vi "CvrtCell2Data.vi"(8 "error in (no error)":errorcluster, 9 "ge_HdrNames":T1, 10 "Item Name":string, 11 "RTD in":refnum<class "RTD.lvclass">) -> (0 "error out":errorcluster, 3 "RTD out":refnum<class "RTD.lvclass">)   [LabVIEW 2018, in "Measurement Channels.lvlib" / "RTD.lvclass"]
uses:
  RTD.lvclass
  C:/Users/Jeff Tipps/Documents/DAQMan/source/Classes/Measurements/Class Channel/Channel.lvclass
  Common/Controls/HeaderNames.ctl
  SubVIs Table/Custom Ctls Table/ge_ColType.ctl
  RTD.lvclass/RTD.ctl
  Class Channel/Write Unit_EU.vi
  Class Channel/Channel.lvclass
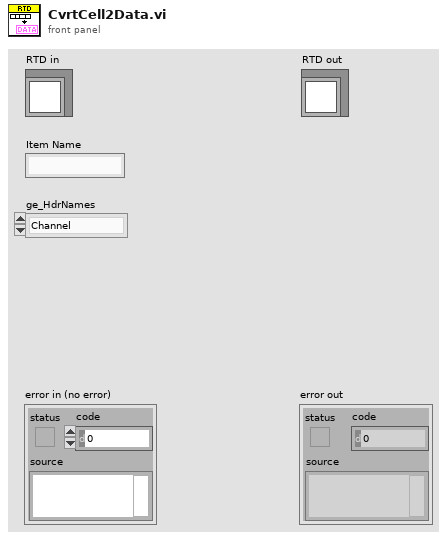
[diagram p1: front panel]
types:
  T1 = typedef "HeaderNames.ctl" = enum16{"Channel", "Device", "Spacer", "Description", "MB", "Range", "Terminal", "Coupling", "Thresh (V)", "Pulse/Rev", "Slope", "Min EU", "Min RPM", "mV/EU", "Iex", "Temp Units", "Type", "CJC Src", "CJC Val", "Ro", "Wire Cfg", "Strain Mode", "Vex", "Bridge Type", "GF", "Gauge Res", "Poisson", "Lead Res", "Init Strain", "GAF", "Scale", "Offset", "Unit (EU)", "dB?", "dB Ref", "Cal Mag", "Cal Units", "Max Temp", "Min Temp", "Max Strain", "Min Strain"}
  T2 = typedef "ge_ColType.ctl" = enum16{"Volts", "Amps", "Ohms", "TermCfg", "WireCfg", "Coup", "Slope", "Iex", "CalUnits", "ThrmUnits", "ThrmType", "CJCSrc", "BrdgType", "Strn Mode", "RTDType"}
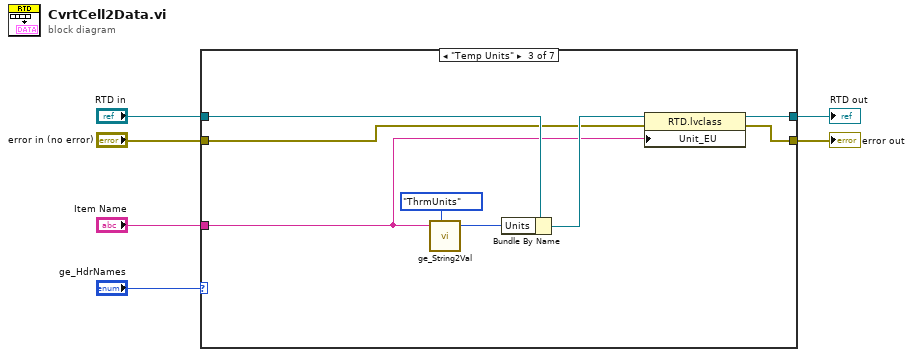
[diagram p0: block diagram]
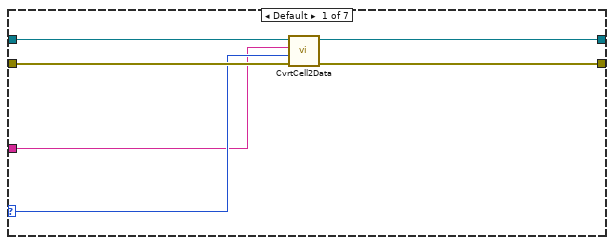
[diagram p2: hidden frame]
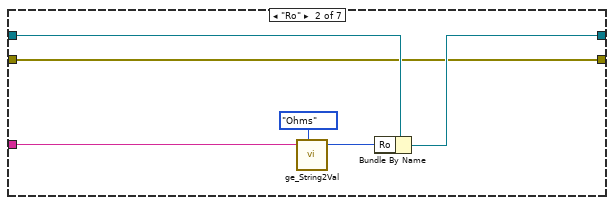
[diagram p3: hidden frame]
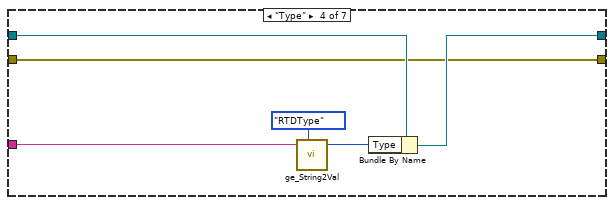
[diagram p4: hidden frame]
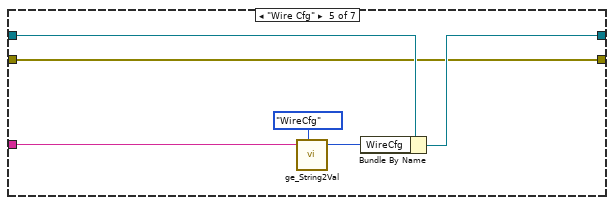
[diagram p5: hidden frame]
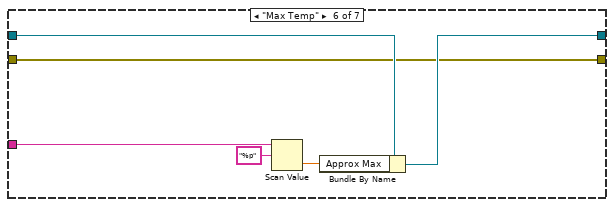
[diagram p6: hidden frame]
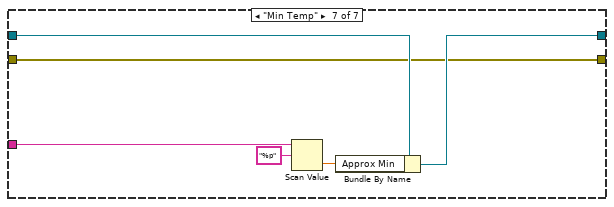
[diagram p7: hidden frame]
diagram:
  n1 = case shown="\"Temp Units\"" "ge_HdrNames" {
    selector: "ge_HdrNames" -> [w10 _ _ _ _ _ _]
    tunnel: "RTD in" -> [w12 w18 w26 w32 w38 w44 w50]
    tunnel: [w8 w17 w23 w31 w37 w43 w49] -> w5
    tunnel: "error in (no error)" -> [w11 w16 w19 w30 w36 w42 w48]
    tunnel: [w7 w16 w20 w30 w36 w42 w48] -> w3
    tunnel: "Item Name" -> [w9 w13 w21 w27 w33 w40 w46]
    frame Default {
      n2 = call-parent "CvrtCell2Data.vi"("error in (no error)"=w11, "Header Names"=w10, "Item Name"=w9, "Channel in"=w12) -> ("error out"=w7:errorcluster, "Channel out"=w8:refnum<class "RTD.lvclass">)  [unwired: 6 in]
    }
    frame "Ro" {
      n3 = call "ge_String2Val.vi"("String"=w13, "ColType"=ge_ColType."Ohms") -> ("Value"=w14:u16)  [unwired: 4 in, 1 out]
      n4 = Bundle By Name(cluster=w18, "Ro"=w14) -> (w17:refnum<class "RTD.lvclass">)
    }
    frame "Temp Units" {
      n5 = call "ge_String2Val.vi"("String"=w21, "ColType"=ge_ColType."ThrmUnits") -> ("Value"=w24:u16)  [unwired: 4 in, 1 out]
      n6 = Bundle By Name(cluster=w26, "Units"=w24) -> (w22:refnum<class "RTD.lvclass">)
      n7 = property class="RTD.lvclass"(reference=w22, error in=w19, "Unit_EU"=w21) -> (reference out=w23:refnum<class "RTD.lvclass">, error out=w20:errorcluster)
    }
    frame "Type" {
      n8 = call "ge_String2Val.vi"("String"=w27, "ColType"=ge_ColType."RTDType") -> ("Value"=w28:u16)  [unwired: 4 in, 1 out]
      n9 = Bundle By Name(cluster=w32, "Type"=w28) -> (w31:refnum<class "RTD.lvclass">)
    }
    frame "Wire Cfg" {
      n10 = call "ge_String2Val.vi"("String"=w33, "ColType"=ge_ColType."WireCfg") -> ("Value"=w34:u16)  [unwired: 4 in, 1 out]
      n11 = Bundle By Name(cluster=w38, "WireCfg"=w34) -> (w37:refnum<class "RTD.lvclass">)
    }
    frame "Max Temp" {
      n12 = Scan Value(string=w40, format string="%p") -> (value=w39:dbl)  [unwired: 1 in, 1 out]
      n13 = Bundle By Name(cluster=w44, "Approx Max"=w39) -> (w43:refnum<class "RTD.lvclass">)
    }
    frame "Min Temp" {
      n14 = Scan Value(string=w46, format string="%p") -> (value=w45:dbl)  [unwired: 1 in, 1 out]
      n15 = Bundle By Name(cluster=w50, "Approx Min"=w45) -> (w49:refnum<class "RTD.lvclass">)
    }
  }
  "error out" <- w3
  "RTD out" <- w5
